vi "Teleop.vi"(10 "Match Info":T1={"Autonomous Elapsed Seconds"=0.0, "TeleOp Elapsed Seconds"=0.0, "Disabled Elapsed Seconds"=0.0, "Visited Autonomous"=FALSE, "Visited TeleOp"=FALSE, "Visited Disabled"=FALSE, "Autonomous Settings"={"Autonomous Style"=enum."Independent", "VI Refnum"=refnum}}, 11 "Call Context":T2) -> ()   [LabVIEW 2017]
doc: "This VI is called for each TeleOp packet received from the DS where the robot is not disabled. It is often used to read from the joysticks and update I/O or to update setpoints for timed control loops. It should complete and return within 20 milliseconds or it may miss DS packets."
uses:
  <vilib>/Rock Robotics/WPI/DriverStation/WPI_DriverStationDerivedRobotMode.ctl
  <vilib>/Rock Robotics/WPI/DriverStation/WPI_DriverStationMatch Info.ctl
  SwerveLibrary/Controllers.ctl
  <vilib>/Rock Robotics/WPI/Utilities/WPI_GetSetVariantRefNum.vi
  Robot Global Data.vi
  SwerveLibrary/Huskie Swerve.lvlib
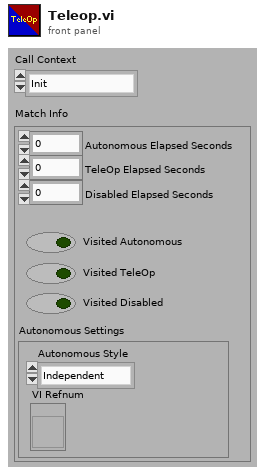
[diagram p1: front panel]
types:
  T1 = typedef "WPI_DriverStationMatch Info.ctl" = cluster{"Autonomous Elapsed Seconds":dbl, "TeleOp Elapsed Seconds":dbl, "Disabled Elapsed Seconds":dbl, "Visited Autonomous":bool, "Visited TeleOp":bool, "Visited Disabled":bool, "Autonomous Settings":cluster{"Autonomous Style":enum16{"Iterative", "Independent"}, "VI Refnum":refnum<vi>}}
  T2 = typedef "WPI_DriverStationDerivedRobotMode.ctl" = enum16{"Init", "Execute", "Stop"}
  T3 = cluster{"X":dbl, "Y":dbl, "Z":dbl, "X Drive":bool, "Field Relative":bool, "Actuate Grabber":bool, "Inverse Drive":bool}
  T4 = typedef "Huskie Swerve.lvlib/Controllers.ctl" = enum16{"Joystick", "Buttons"}
  T5 = typedef "WPI_JoystickDevRef.ctl" = cluster{"Device":T6}
  T6 = typedef "WPI_JoystickDeviceEnum.ctl" = enum16{"USB 0", "USB 1", "USB 2", "USB 3", "USB 4", "USB 5"}
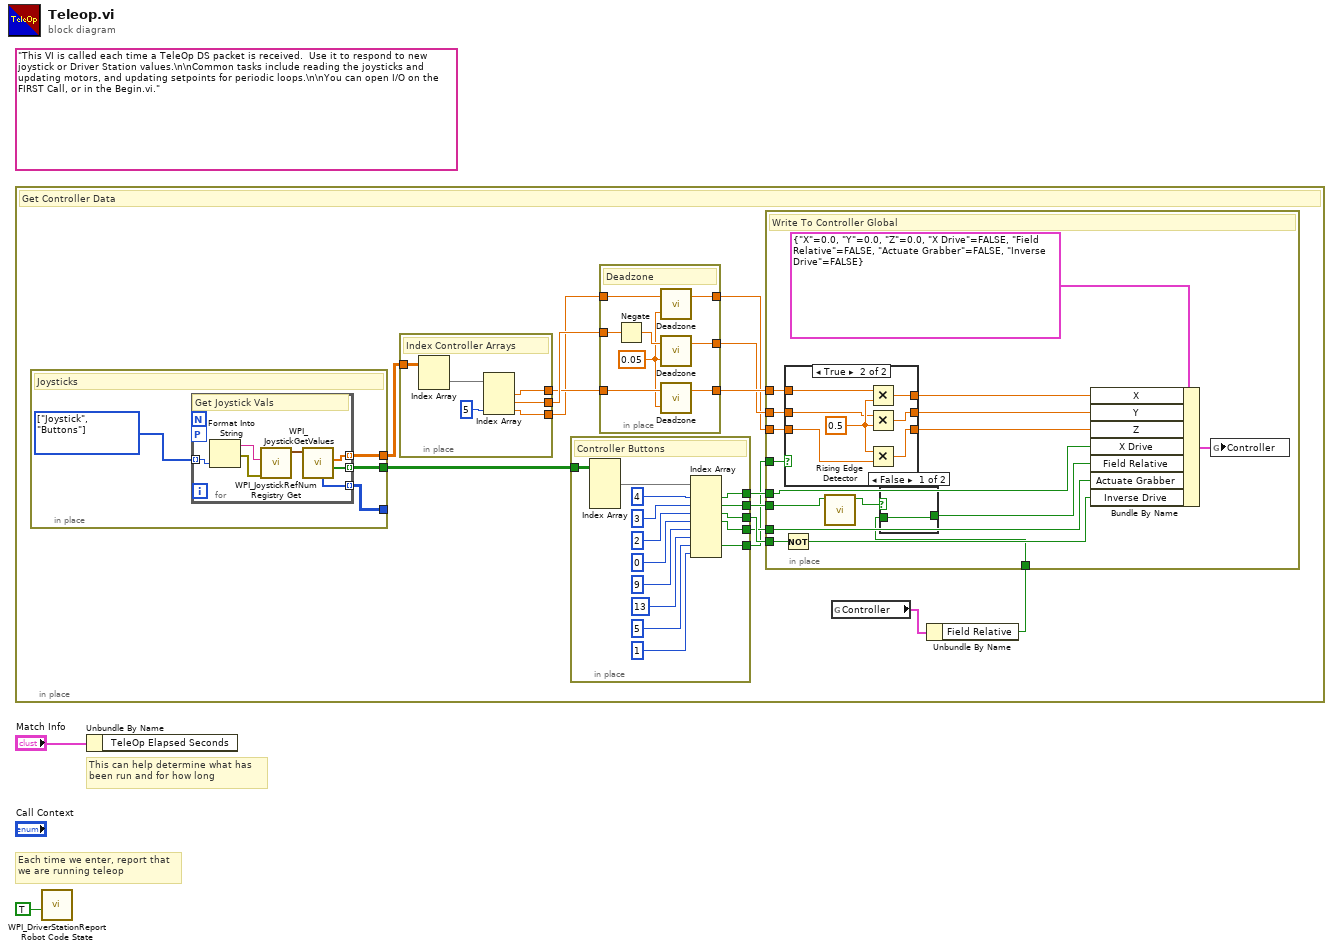
[diagram p0: block diagram]
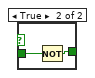
[diagram p2: hidden frame]
diagram:
  (unwired) "This VI is called each time a TeleOp DS packet is received.  Use it to respond to new joystick or Driver Station values.\n\nCommon tasks include reading the joysticks and updating motors, and updating setpoints for periodic loops.\n\nYou can open I/O on the FIRST Call, or in the Begin.vi."
  # "Each time we enter, report that\nwe are running teleop"
  # "This can help determine what has\nbeen run and for how long"
  n1 = in-place "In Place Element Structure" {
    # "Get Controller Data"
    n2 = in-place {
      in-place-border: [w66] -> w17
      in-place-border: [w65] -> w10
      in-place-border: [w64] -> _
      w63 = T4[] [enum."Joystick", enum."Buttons"] items=["Joystick", "Buttons"] ("Array")
      # "Joysticks"
      n3 = for {
        workers-P: _ -> [_]
        tunnel: w63 -> [w67] mode=indexing
        tunnel: [w72] -> w66 mode=indexing
        tunnel: [w71] -> w65 mode=indexing
        tunnel: [w70] -> w64 mode=indexing
        # "Get Joystick Vals"
        n4 = Format Into String(w67) -> (resulting string=w68:string, error out=w69:errorcluster)  [unwired: 3 in]
        n5 = call <vilib>:"WPI_JoystickRefNum Registry Get.vi"("error in (no error)"=w69, "refnum name"=w68) -> ("JoystickDevRef"=w73:T5)  [unwired: 8 in, 1 out]
        n6 = call <vilib>:"WPI_JoystickGetValues.vi"("JoystickDevRef"=w73) -> ("Buttons"=w71:bool[], "Axes"=w72:dbl[], "POVs"=w70:i16[])  [unwired: 6 in, 2 out]
      }
    }
    n7 = in-place {
      in-place-border: w17 -> [w87]
      in-place-border: [w84] -> w16
      in-place-border: [w83] -> w15
      in-place-border: [w82] -> w11
      # "Index Controller Arrays"
      n8 = Index Array(array=w87) -> (element=w86:dbl[])  [unwired: 2 in]
      n9 = Index Array(array=w86, index #3=5) -> (element #1=w83:dbl, element #2=w84:dbl, element #3=w82:dbl)  [unwired: 2 in]
    }
    n10 = in-place {
      in-place-border: w10 -> [w62]
      in-place-border: [w59] -> w9
      in-place-border: [w57] -> w8
      in-place-border: [w55] -> w7
      in-place-border: [w53] -> w6
      in-place-border: [w49] -> w5
      # "Controller Buttons"
      n11 = Index Array(array=w62) -> (element #1=w61:bool[])  [unwired: 4 in, 1 out]
      n12 = Index Array(array=w61, index #1=4, index #2=3, index #3=2, index #4=0, index #5=9 ("index"), index #6=13 ("index"), index #7=5 ("index"), index #8=1 ("index")) -> (element #1=w59:bool, element #2=w57:bool, element #3=w55:bool, element #4=w53:bool, element #7=w49:bool)  [unwired: 3 out]
    }
    n13 = in-place {
      in-place-border: w16 -> [w80]
      in-place-border: w15 -> [w79]
      in-place-border: [w77] -> w14
      in-place-border: [w76] -> w13
      in-place-border: [w75] -> w12
      in-place-border: w11 -> [w74]
      w78 = 0.05
      # "Deadzone"
      n14 = Negate(x=w80) -> (-x=w81:dbl)
      n15 = call "Deadzone.vi"("Deadzone"=w78, "Value"=w74) -> ("Numeric"=w75:dbl)  [unwired: 1 out]
      n16 = call "Deadzone.vi"("Deadzone"=w78, "Value"=w81) -> ("Numeric"=w76:dbl)  [unwired: 1 out]
      n17 = call "Deadzone.vi"("Deadzone"=w78, "Value"=w79) -> ("Numeric"=w77:dbl)  [unwired: 1 out]
    }
    n18 = global read "Robot Global Data.vi" "Controller"() -> (w4:T3)
    n19 = Unbundle By Name(w4) -> ("Field Relative"=w3:bool)
    n20 = in-place {
      in-place-border: w14 -> [w29]
      in-place-border: w13 -> [w26]
      in-place-border: w12 -> [w24]
      in-place-border: w9 -> [w33]
      in-place-border: w8 -> [w30]
      in-place-border: w7 -> [w32]
      in-place-border: w6 -> [w31]
      in-place-border: w5 -> [w27]
      in-place-border: w3 -> [w19]
      # "Write To Controller Global"
      n21 = Not(x=w32) -> (.not. x?=w22:bool)
      n22 = case shown="True" w27 {
        tunnel: w29 -> [w40 w43]
        tunnel: [w40 w44] -> w28
        tunnel: w26 -> [w39 w46]
        tunnel: [w39 w45] -> w25
        tunnel: w24 -> [w38 w42]
        tunnel: [w38 w41] -> w23
        frame False {
        }
        frame True {
          w47 = 0.5
          n23 = Multiply(x=w43, y=w47) -> (x*y=w44:dbl)
          n24 = Multiply(x=w46, y=w47) -> (x*y=w45:dbl)
          n25 = Multiply(x=w47, y=w42) -> (x*y=w41:dbl)
        }
      }
      n26 = call "Rising Edge Detector.vi"("Input"=w30) -> ("Rising edge?"=w20:bool)  [unwired: 10 in]
      n27 = case shown="False" w20 {
        tunnel: w19 -> [w35 w36]
        tunnel: [w35 w37] -> w18
        frame False {
        }
        frame True {
          n28 = Not(x=w36) -> (.not. x?=w37:bool)
        }
      }
      n29 = Bundle By Name(cluster=T3 {"X"=0.0, "Y"=0.0, "Z"=0.0, "X Drive"=FALSE, "Field Relative"=FALSE, "Actuate Grabber"=FALSE, "Inverse Drive"=FALSE}, "X"=w28, "Y"=w25, "Z"=w23, "X Drive"=w33, "Field Relative"=w18, "Actuate Grabber"=w31, "Inverse Drive"=w22) -> (w21:T3)
      n30 = global write "Robot Global Data.vi" "Controller"(w21) -> ()
    }
  }
  n31 = call <vilib>:"WPI_DriverStationReport Robot Code State.vi"("TeleOp"=TRUE ("Autonomous")) -> ()  [unwired: 10 in, 1 out]
  n32 = Unbundle By Name("Match Info") -> ()  [unwired: 1 out]
